vi "NTP.vi"() -> ()   [LabVIEW 2023]
uses:
  <vilib>/Utility/file.llb/Write Delimited Spreadsheet (I64).vi
panel:
  out "file path (Check data file)":path=path "/Users/blagojnikolov/Desktop/@tmp/checkRes.txt"
  in  "Time Stop":bool
  out "appended array":string[](array[string])
  out "Average in row":u64[](array[numeric]) format="%-2.0f"
  out "Deviation by row":i64[][](array[numeric])
  in  "Last Draw":i64[](array[numeric])
  out "Matches":i64[][](array[numeric])
  out "Matches":i32[](array[numeric])
  out "Last Suppose":i32[][](array[numeric])
  out "?":bool
  in  "Deviation":bool
  in  "Check":bool
  in  "Play":bool
  out "Your Suppose":i32[][](array[numeric])
  out "Waveform Chart":i64[][](graph)
  in  "Stop":bool
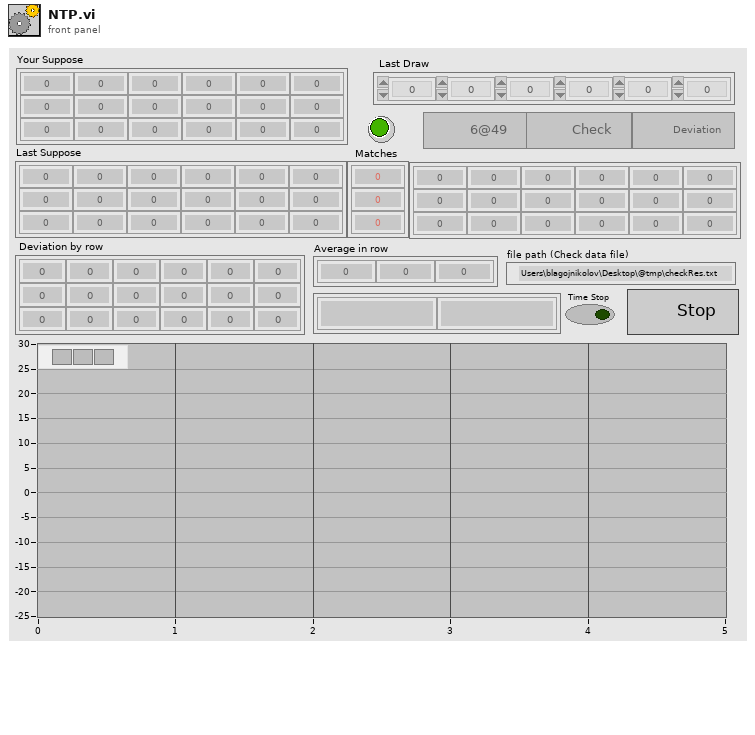
[diagram p1: front panel]
types:
  T1 = enum8{"Enabled", "Disabled", "Disabled and Grayed Out"}
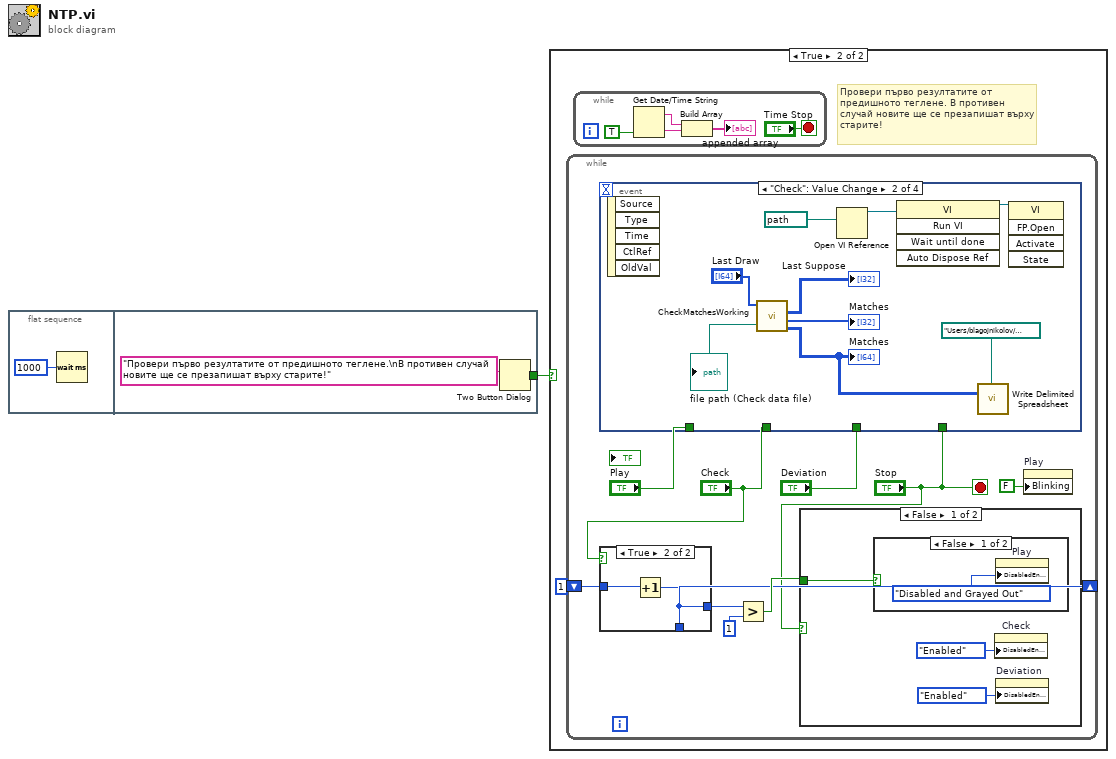
[diagram p0: block diagram]
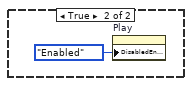
[diagram p4: hidden frame]
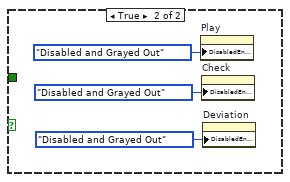
[diagram p5: hidden frame]
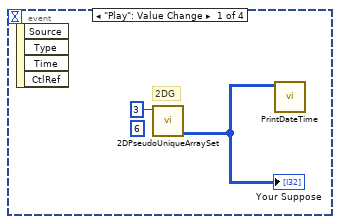
[diagram p6: hidden frame]
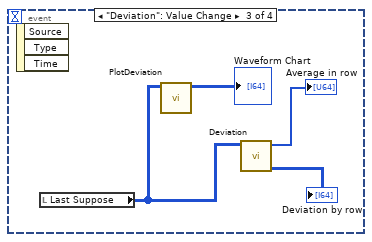
[diagram p7: hidden frame]
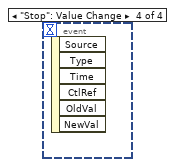
[diagram p8: hidden frame]
diagram:
  n1 = flat-sequence {
    tunnel: [w3] -> w1
    frame #0 {
      n2 = Wait (ms)(milliseconds to wait=u32 1000) -> ()  [unwired: 1 out]
    }
    frame #1 {
      n3 = Two Button Dialog(message="Провери първо резултатите от предишното теглене.\nВ противен случай новите ще се презапишат върху старите!") -> (T button?=w3:bool)  [unwired: 2 in]
    }
  }
  n4 = case shown="True" w1 {
    frame False {
    }
    frame True {
      # "Провери първо резултатите от \nпредишното теглене. В противен случай новите ще се презапишат върху старите!"
      n5 = while {
        shift-right: [w13] -> _
        shift-left: i64 1 -> [w15]
        stop <- "Stop" stop-if-true
        n6 = event shown="[1] \"Check\": Value Change" {
          selector: _ -> [_ _ _ _]
          dyn-events: _ -> [_ _ _ _]
          timeout: _ -> [_ _ _ _]
          tunnel: "Play" -> [_ _ _ _]
          tunnel: "Check" -> [_ _ _ _]
          tunnel: "Deviation" -> [_ _ _ _]
          tunnel: "Stop" -> [_ _ _ _]
          event "Play": Value Change {
            (unwired) 6 ("Colums")
            # "2DG"
            n7 = event-data() -> ()  [unwired: 1 in, 4 out]
            n8 = call "2DPseudoUniqueArraySet.vi"("Rows"=3) -> ("2D Double Array"=w32:i32[][])  [unwired: 9 in, 1 out]
            "Your Suppose" <- w32
            n9 = call "PrintDateTime.vi"("2D Double"=w32) -> ()  [unwired: 10 in, 1 out]
          }
          event "Check": Value Change {
            n10 = event-data() -> ()  [unwired: 1 in, 5 out]
            n11 = call "CheckMatchesWorking.vi"("Последен тираж"="Last Draw") -> (0:w35:i64[][], "Съвпадения"=→"Matches":i32[], "Залози"=→"Last Suppose":i32[][], "file path (dialog if empty)"=→"file path (Check data file)":path)  [unwired: 7 in]
            "Matches" <- w35
            n12 = Open VI Reference(vi path=path "/Users/blagojnikolov/Library/Mobile Documents/com~apple~CloudDocs/» LabView/LabView/Project'24/Projects/649/subVI Tools/CollorCellsInTableOnly.vi") -> (vi reference=w37:refnum<vi>)  [unwired: 5 in, 1 out]
            n13 = invoke class="VI" method="Run VI"(reference=w37) -> (reference out=w36:refnum<vi>)  [unwired: 4 in, 4 out]
            n14 = call-poly <vilib>:"Write Delimited Spreadsheet.vi"("file path (dialog if empty)"=path "/Users/blagojnikolov/Desktop/@tmp/matches.txt", "2D data"=w35) -> ()  [unwired: 12 in, 2 out]
            n15 = invoke class="VI" method="FP.Open"(reference=w36) -> ()  [unwired: 4 in, 5 out]
          }
          event "Deviation": Value Change {
            n16 = event-data() -> ()  [unwired: 1 in, 3 out]
            n17 = local read "Last Suppose"() -> (w44:i32[][])
            n18 = call "PlotDeviation.vi"("Array"=w44) -> ("Waveform Chart"=→"Waveform Chart":i64[][])  [unwired: 8 in, 2 out]
            n19 = call "Deviation.vi"("2D  Array"=w44) -> ("Deviation by row"=→"Deviation by row":i64[][], "Average in row"=→"Average in row":u64[])  [unwired: 9 in]
          }
          event "Stop": Value Change {
            n20 = event-data() -> ()  [unwired: 1 in, 6 out]
          }
        }
        n21 = case shown="True" "Check" {
          tunnel: [w21 w22] -> w14
          tunnel: [w21 w22] -> w13
          tunnel: w15 -> [w21 w23]
          frame False {
          }
          frame True {
            n22 = Increment(x=w23) -> (x+1=w22:i64)
          }
        }
        n23 = Greater?(x=w14, y=i64 1) -> (0:w16:bool)
        n24 = case shown="False" "Stop" {
          tunnel: w16 -> [w24 _]
          frame False {
            n25 = case shown="False" w24 {
              frame False {
                n26 = property on="Play" class="Bool"("DisabledEnum"=T1."Disabled and Grayed Out" ("Disabled")) -> ()  [unwired: 2 in, 2 out]
              }
              frame True {
                n27 = property on="Play" class="Bool"("DisabledEnum"=T1."Enabled" ("Disabled")) -> ()  [unwired: 2 in, 2 out]
              }
            }
            n28 = property on="Check" class="Bool"("DisabledEnum"=T1."Enabled" ("Disabled")) -> ()  [unwired: 2 in, 2 out]
            n29 = property on="Deviation" class="Bool"("DisabledEnum"=T1."Enabled" ("Disabled")) -> ()  [unwired: 2 in, 2 out]
          }
          frame True {
            n30 = property on="Play" class="Bool"("DisabledEnum"=T1."Disabled and Grayed Out" ("Disabled")) -> ()  [unwired: 2 in, 2 out]
            n31 = property on="Check" class="Bool"("DisabledEnum"=T1."Disabled and Grayed Out" ("Disabled")) -> ()  [unwired: 2 in, 2 out]
            n32 = property on="Deviation" class="Bool"("DisabledEnum"=T1."Disabled and Grayed Out" ("Disabled")) -> ()  [unwired: 2 in, 2 out]
          }
        }
        n33 = property on="Play" class="Bool"("Blinking"=FALSE) -> ()  [unwired: 2 in, 2 out]
      }
      n34 = while {
        stop <- "Time Stop" stop-if-true
        n35 = Get Date/Time String(want seconds? (F)=TRUE) -> (date string=w10:string, time string=w9:string)  [unwired: 2 in]
        n36 = Build Array(w10, w9) -> (→"appended array":string[])
      }
    }
  }
